vi "CSVsub_ConditionalDataCheck.vi"(6 "index in":i32, 8 "error in":errorcluster, 9 "A[Data]":string[](array[string]), 10 "A[Labels]":string[](array[string]), 11 "Data":string[][](array[string])) -> (0 "error out":errorcluster, 2 "Headers":string[](array[string]), 3 "Data Index":i32[](array[numeric]))   [LabVIEW 2014, in "TableLogger_CSV_Actor.lvlib" / "TableLogger_CSV_Actor.lvclass"]
uses:
  TableLogger_CSV_Actor.lvclass
  <userlib>/_OpenG.lib/array/array.llb/Search 1D Array (String)__ogtk.vi
  <userlib>/_OpenG.lib/array/array.llb/Search 1D Array (I32)__ogtk.vi
  <userlib>/_OpenG.lib/array/array.llb/Index 1D Array Elements (I32)__ogtk.vi
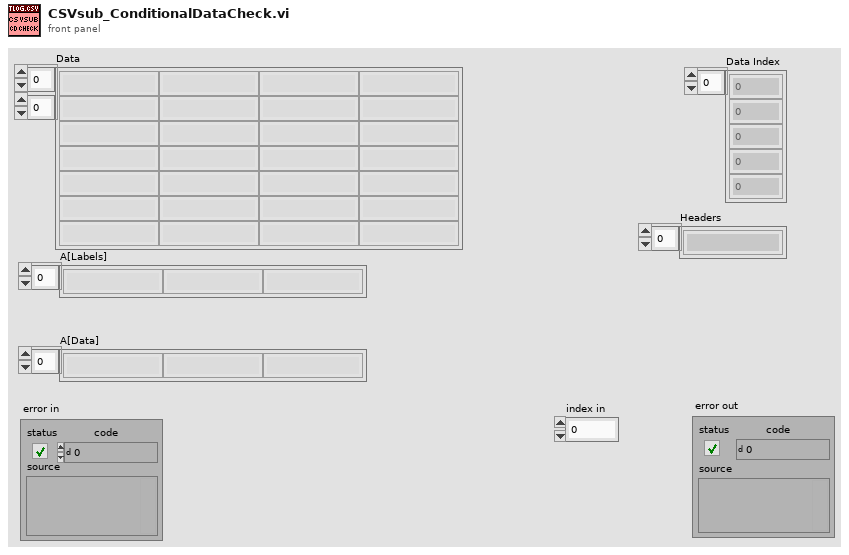
[diagram p1: front panel]
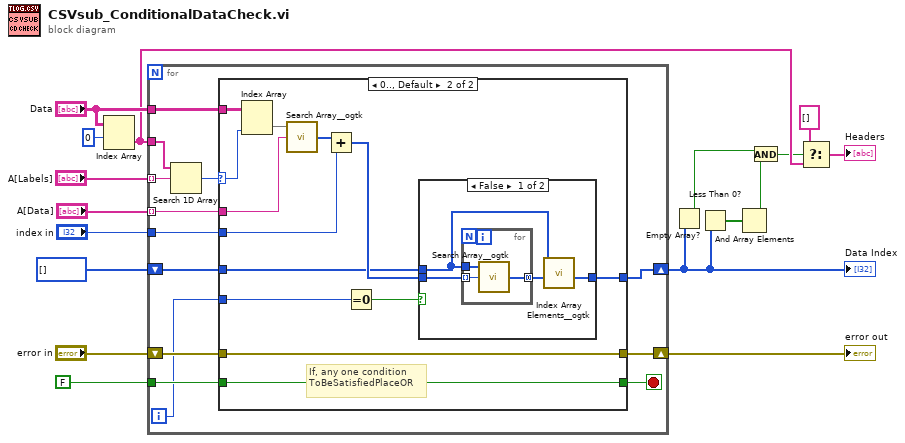
[diagram p0: block diagram]
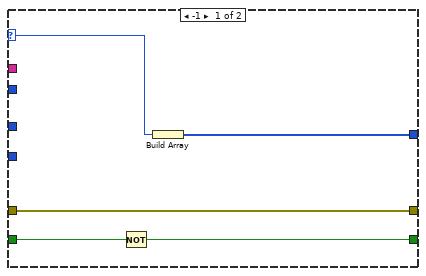
[diagram p2: hidden frame]
diagram:
  n1 = Index Array(array="Data", index (row)=0) -> (element=w8:string[])  [unwired: 1 in]
  n2 = for {
    tunnel: "A[Labels]" -> [w30] mode=indexing
    tunnel: "A[Data]" -> [w29] mode=indexing
    tunnel: "Data" -> [w27]
    tunnel: w8 -> [w26]
    shift-right: [w23] -> w11
    shift-left: "error in" -> [w22]
    tunnel: "index in" -> [w25]
    tunnel: FALSE -> [w28]
    shift-right: [w20] -> w3
    shift-left: i32[] [] -> [w19]
    i -> [w18]
    stop <- w21 stop-if-true
    n3 = Search 1D Array(1D array=w26, element=w30) -> (index of element=w24:i32)  [unwired: 1 in]
    n4 = case shown="0.., Default" w24 {
      selector: w24 -> [w32 w47]
      tunnel: w27 -> [_ w48]
      tunnel: w29 -> [_ w44]
      tunnel: w28 -> [w34 w42]
      tunnel: w25 -> [_ w43]
      tunnel: [w35 w46] -> w23
      tunnel: w22 -> [w35 w46]
      tunnel: [w33 w42] -> w21
      tunnel: [w31 w39] -> w20
      tunnel: w19 -> [_ w38]
      tunnel: w18 -> [_ w36]
      frame -1 {
        n5 = Not(x=w34) -> (.not. x?=w33:bool)
        n6 = Build Array(w32) -> (w31:i32[])
      }
      frame 0.., Default {
        # "If, any one condition ToBeSatisfiedPlaceOR"
        n7 = Index Array(array=w48, index (col)=w47) -> (element=w45:string[])  [unwired: 1 in]
        n8 = call-poly <userlib>:"Search Array__ogtk.vi"("Array"=w45, "Element Data"=w44) -> ("Indices of Elements"=w41:i32[])  [unwired: 7 in]
        n9 = Add(x=w41, y=w43) -> (x+y=w40:i32[])
        n10 = Equal To 0?(x=w36) -> (x = 0?=w37:bool)
        n11 = case shown="False" w37 {
          tunnel: w40 -> [w51 w56]
          tunnel: [w50 w56] -> w39
          tunnel: w38 -> [w49 _]
          frame False {
            n12 = for {
              tunnel: w49 -> [w55]
              tunnel: w51 -> [w54] mode=indexing
              tunnel: [w53] -> w52 mode=concatenating
              n13 = call-poly <userlib>:"Search Array__ogtk.vi"("Array"=w55, "Element Data"=w54) -> ("Indices of Elements"=w53:i32[])  [unwired: 7 in]
            }
            n14 = call-poly <userlib>:"Index Array Elements__ogtk.vi"("indices"=w52, "array"=w49) -> ("elements"=w50:i32[])  [unwired: 9 in]
          }
          frame True {
          }
        }
      }
    }
  }
  "Data Index" <- w3
  "error out" <- w11
  n15 = Empty Array?(array=w3) -> (empty?=w4:bool)
  n16 = Less Than 0?(x=w3) -> (x < 0?=w2:bool[])
  n17 = And Array Elements(Boolean array=w2) -> (logical AND=w1:bool)
  n18 = And(x=w4, y=w1) -> (x .and. y?=w5:bool)
  n19 = Select(t=string[] [], s=w5, f=w8) -> (s? t:f=→"Headers":string[])
